vi "Calculate Absolute Max Value.vi"(10 "Data":dbl[](array[numeric])) -> (1 "Abs max index":i32, 3 "Abs max value":dbl)   [LabVIEW 2021, in "Linearity_DAC.lvlib"]
uses:
  Linearity_DAC.lvlib
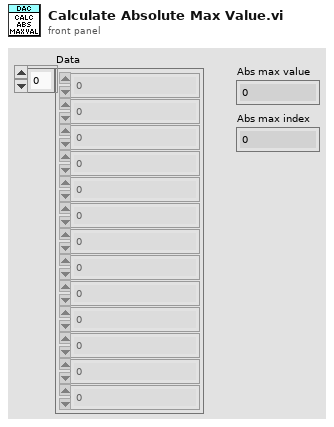
[diagram p1: front panel]
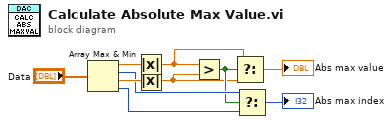
[diagram p0: block diagram]
diagram:
  n1 = Array Max & Min(array="Data") -> (max value=w9:dbl, max index (indices)=w7:i32, min value=w8:dbl, min index (indices)=w6:i32)
  n2 = Absolute Value(x=w9) -> (abs(x)=w2:dbl)
  n3 = Absolute Value(x=w8) -> (abs(x)=w1:dbl)
  n4 = Greater?(x=w2, y=w1) -> (0:w5:bool)
  n5 = Select(t=w2, s=w5, f=w1) -> (s? t:f=→"Abs max value":dbl)
  n6 = Select(t=w7, s=w5, f=w6) -> (s? t:f=→"Abs max index":i32)
